vi "Elapsed Timer.vi"(10 "Reset":bool caption="리셋", 11 "Time Target (s)":dbl=2.0) -> (2 "Time has Elapsed":bool, 3 "Elapsed Time (s)":dbl)   [LabVIEW 2018]
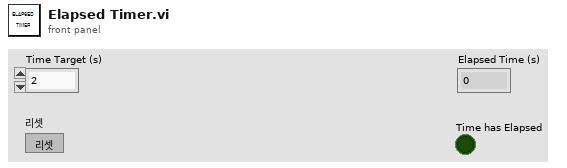
[diagram p1: front panel]
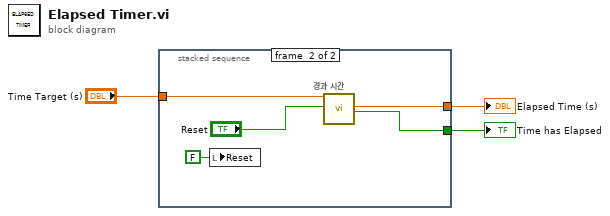
[diagram p0: block diagram]
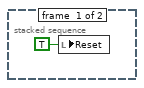
[diagram p2: hidden frame]
diagram:
  n1 = stacked-sequence {
    tunnel: "Time Target (s)" -> [_ w9]
    tunnel: [_ w6] -> w2
    tunnel: [_ w5] -> w1
    frame #0 {
      n2 = local write "Reset"(TRUE ("Reset")) -> ()
    }
    frame #1 {
      n3 = local write "Reset"(FALSE ("Reset")) -> ()
      n4 = call "경과 시간"("Time Target (s)"=w9, "Reset"="Reset") -> ("Elapsed Time (s)"=w5:dbl, "Time has Elapsed"=w6:bool)  [unwired: 10 in, 6 out]
    }
  }
  "Time has Elapsed" <- w2
  "Elapsed Time (s)" <- w1
